vi "Control Panel Values Changed.vi"(8 "error in (no error)":errorcluster, 9 "Old data":variant, 10 "New data":variant, 11 "Neocera LTC-21 in":refnum<class "Neocera LTC-21.lvclass">) -> (0 "error out":errorcluster, 3 "Neocera LTC-21 out":refnum<class "Neocera LTC-21.lvclass">)   [LabVIEW 2015, in "Neocera LTC-21.lvclass"]
uses:
  Neocera LTC-21.lvclass
  Neocera Front Panel Data.ctl
  Neocera Heater Ranges.ctl
  Neocera Set Point Aproach.ctl
  Instrument/Read VISA Resource.vi
  Instrument/Write VISA Resource.vi
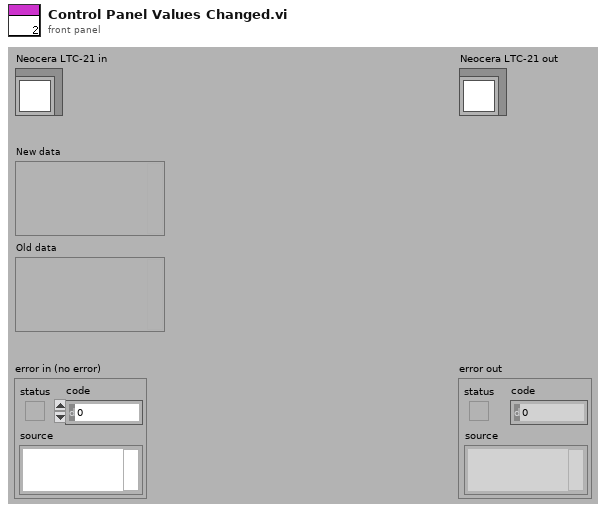
[diagram p1: front panel]
types:
  T1 = typedef "Neocera Front Panel Data.ctl" = cluster{"Channels to measure":dbl[], "Record heater":bool, "Set point":dbl, "Set Heater Range":T2, "Control":bool, "Approach":T3, "Ramp rate, K/min":dbl, "Control Channel":i16, "P":dbl, "I":dbl, "D":dbl, "Suspend heater":bool}
  T2 = typedef "Neocera Heater Ranges.ctl" = enum16{"Off", "0.05W", "0.5W", "5W", "50W"}
  T3 = typedef "Neocera Set Point Aproach.ctl" = enum16{"Instant", "Ramp"}
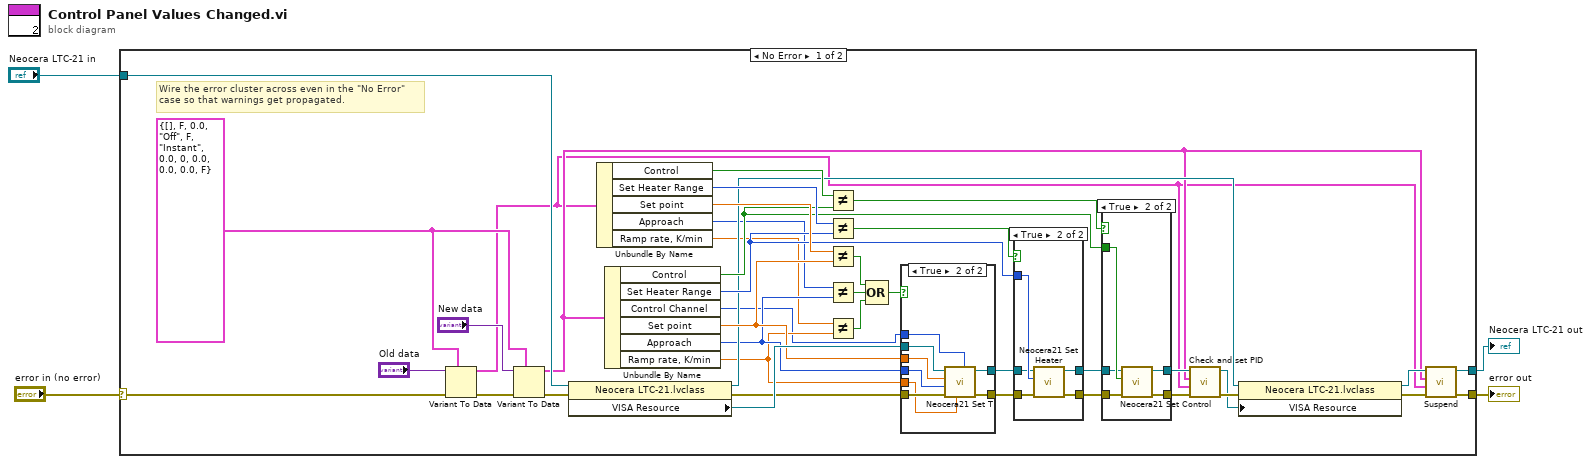
[diagram p0: block diagram]
diagram:
  n1 = case shown="No Error" "error in (no error)" {
    selector: "error in (no error)" -> [w34 w71]
    tunnel: [w9 w71] -> w3
    tunnel: [w11 w70] -> w1
    tunnel: "Neocera LTC-21 in" -> [w33 w70]
    frame No Error {
      w43 = T1 {"Channels to measure"=[], "Record heater"=FALSE, "Set point"=0.0, "Set Heater Range"=enum."Off", "Control"=FALSE, "Approach"=enum."Instant", "Ramp rate, K/min"=0.0, "Control Channel"=0, "P"=0.0, "I"=0.0, "D"=0.0, "Suspend heater"=FALSE} ("Front Panel Data")
      # "Wire the error cluster across even in the \"No Error\"\ncase so that warnings get propagated."
      n2 = Variant To Data(error in=w34, type=w43, Variant="Old data") -> (data=w7:T1, error out=w45:errorcluster)
      n3 = Variant To Data(error in=w45, type=w43, Variant="New data") -> (data=w8:T1, error out=w40:errorcluster)
      n4 = property class="Neocera LTC-21.lvclass"(reference=w33, error in=w40) -> (reference out=w22:refnum<class "Neocera LTC-21.lvclass">, error out=w39:errorcluster, "VISA Resource"=w41:refnum<visa-resource-name>)
      n5 = Unbundle By Name(w7) -> ("Control"=w30:bool, "Set Heater Range"=w37:T2, "Set point"=w42:dbl, "Approach"=w21:T3, "Ramp rate, K/min"=w19:dbl)
      n6 = Unbundle By Name(w8) -> ("Control"=w24:bool, "Set Heater Range"=w25:T2, "Control Channel"=w14:i16, "Set point"=w26:dbl, "Approach"=w20:T3, "Ramp rate, K/min"=w18:dbl)
      n7 = Not Equal?(x=w30, y=w24) -> (x != y?=w32:bool)
      n8 = Not Equal?(x=w37, y=w25) -> (x != y?=w38:bool)
      n9 = Not Equal?(x=w42, y=w26) -> (x != y?=w44:bool)
      n10 = Not Equal?(x=w21, y=w20) -> (x != y?=w16:bool)
      n11 = Not Equal?(x=w19, y=w18) -> (x != y?=w15:bool)
      n12 = Compound Arithmetic op=OR(w44, w16, w15) -> (w17:bool)
      n13 = case shown="True" w17 {
        tunnel: w39 -> [w61 w69]
        tunnel: [w61 w68] -> w36
        tunnel: w26 -> [_ w65]
        tunnel: w41 -> [w60 w66]
        tunnel: [w60 w67] -> w35
        tunnel: w20 -> [_ w64]
        tunnel: w18 -> [_ w63]
        tunnel: w14 -> [_ w62]
        frame False {
        }
        frame True {
          n14 = call "Neocera21 Set T.vi"("Channel"=w62, "Ramp rate, K/min"=w63, "error in (no error)"=w69, "Approach"=w64, "Set T"=w65, "VISA Resource Name"=w66) -> ("error out"=w68:errorcluster, "VISA Resource Name Out"=w67:refnum<visa-resource-name>)  [unwired: 4 in]
        }
      }
      n15 = case shown="True" w38 {
        tunnel: w36 -> [w54 w59]
        tunnel: [w54 w57] -> w31
        tunnel: w25 -> [_ w58]
        tunnel: [w53 w56] -> w29
        tunnel: w35 -> [w53 w55]
        frame False {
        }
        frame True {
          n16 = call "Neocera21 Set Heater.vi"("error in (no error)"=w59, "Set T"=w58, "VISA Resource Name"=w55) -> ("error out"=w57:errorcluster, "VISA Resource Name Out"=w56:refnum<visa-resource-name>)  [unwired: 7 in]
        }
      }
      n17 = case shown="True" w32 {
        tunnel: w31 -> [w47 w52]
        tunnel: [w47 w50] -> w23
        tunnel: w24 -> [_ w51]
        tunnel: [w46 w49] -> w13
        tunnel: w29 -> [w46 w48]
        frame False {
        }
        frame True {
          n18 = call "Neocera21 Set Control.vi"("error in (no error)"=w52, "Control"=w51, "VISA Resource Name"=w48) -> ("error out"=w50:errorcluster, "VISA Resource Name Out"=w49:refnum<visa-resource-name>)  [unwired: 7 in]
        }
      }
      n19 = call "Check and set PID.vi"("Error In"=w23, "Old data"=w7, "New data"=w8, "VISA resource name"=w13) -> ("Error Out"=w6:errorcluster, "VISA resource name out"=w5:refnum<visa-resource-name>)  [unwired: 6 in]
      n20 = property class="Neocera LTC-21.lvclass"(reference=w22, error in=w6, "VISA Resource"=w5) -> (reference out=w12:refnum<class "Neocera LTC-21.lvclass">, error out=w10:errorcluster)
      n21 = call "Suspend.vi"("error in (no error)"=w10, "Old data"=w7, "New data"=w8, "Neocera LTC-21 in"=w12) -> ("error out"=w9:errorcluster, "Neocera LTC-21 out"=w11:refnum<class "Neocera LTC-21.lvclass">)  [unwired: 6 in]
    }
    frame Error {
    }
  }
  "error out" <- w3
  "Neocera LTC-21 out" <- w1
